vi "Timed_DeBounce.vi"(1 "Input":bool, 2 "Hold Time(ms)":u32) -> (0 "Output":bool)   [LabVIEW 2017]
uses:
  ArgosLib/Signal Processing/TypeDefs/EdgeDetector_Type.ctl
  ArgosLib/ArgosLib.lvlib
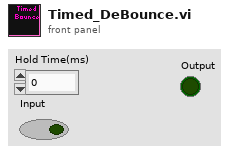
[diagram p1: front panel]
types:
  T1 = typedef "ArgosLib.lvlib/EdgeDetector_Type.ctl" = enum16{"RisingEdge", "FallingEdge", "Both"}
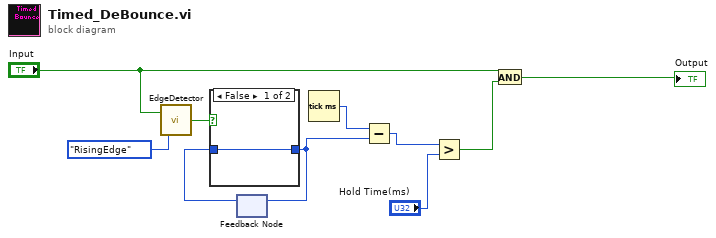
[diagram p0: block diagram]
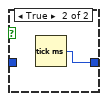
[diagram p2: hidden frame]
diagram:
  n1 = call "EdgeDetector.vi"("DetectorType"=EdgeDetector_Type."RisingEdge", "Input"="Input") -> ("Edge"=w7:bool)
  n2 = feedback #1() -> (w4:u32)  [unwired: 1 in]
  n3 = case shown="False" w7 {
    tunnel: [w11 w12] -> w3
    tunnel: w4 -> [w11 _]
    frame False {
    }
    frame True {
      n4 = Tick Count (ms)() -> (millisecond timer value=w12:u32)
    }
  }
  n5 = feedback-in #1(w3) -> ()
  n6 = Tick Count (ms)() -> (millisecond timer value=w8:u32)
  n7 = Subtract(x=w8, y=w3) -> (x-y=w9:u32)
  n8 = Greater?(x=w9, y="Hold Time(ms)") -> (0:w10:bool)
  n9 = And(x="Input", y=w10) -> (x .and. y?=→"Output":bool)
